vi "get Licor-Source.vi"(0 "Sources":T1[](array[typedef]), 2 "get Source":string(combo), 11 "source data":dbl[](array[numeric])) -> (4 "value":dbl, 8 "Index":i32, 15 "Fehlerkonstante":errorcluster)   [LabVIEW 2010]
uses:
  Licor-Steuerung/LicorLI7000/conventions/Licor-Source.ctl
  Licor-Steuerung/LicorLI7000/LicorLI7000.lvlib
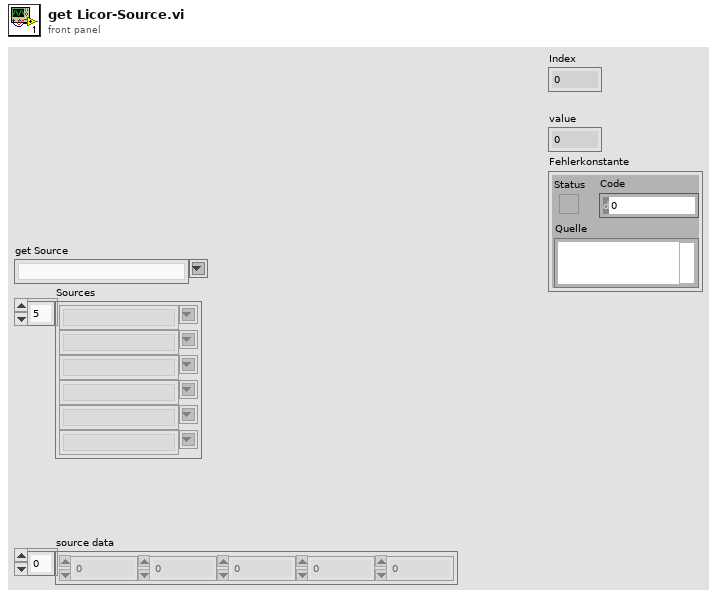
[diagram p1: front panel]
types:
  T1 = typedef "LicorLI7000.lvlib/Licor-Source.ctl" = string
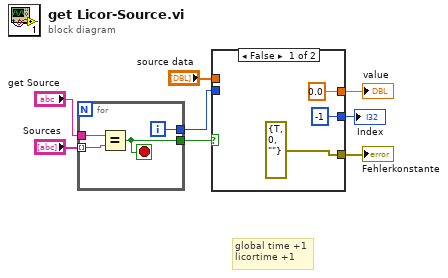
[diagram p0: block diagram]
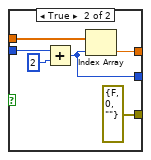
[diagram p2: hidden frame]
diagram:
  # "global time +1\nlicortime +1"
  n1 = for {
    tunnel: "Sources" -> [w12] mode=indexing
    tunnel: "get Source" -> [w11]
    tunnel: [w10] -> w6
    tunnel: [w9] -> w4
    i -> [w9]
    stop <- w10 stop-if-true
    n2 = Equal?(x=w11, y=w12) -> (x = y?=w10:bool)
  }
  n3 = case shown="False" w6 {
    tunnel: "source data" -> [_ w21]
    tunnel: w4 -> [_ w17]
    tunnel: [0.0 ("time (globale Variable)") w20] -> w3
    tunnel: [errorcluster {"status"=TRUE, "code"=0, "source"=""} ("Fehlerkonstante") errorcluster {"status"=FALSE, "code"=0, "source"=""} ("Fehlerkonstante")] -> w2
    tunnel: [-1 w16] -> w1
    frame False {
    }
    frame True {
      n4 = Add(x=w17, y=2) -> (x+y=w16:i32)
      n5 = Index Array(array=w21, index=w16) -> (element=w20:dbl)
    }
  }
  "value" <- w3
  "Fehlerkonstante" <- w2
  "Index" <- w1
